vi "TimebaseSet.vi"(7 "参数查询(0)/设置(1)":bool, 8 "error in (no error)":errorcluster caption="错误输入（无错误）", 9 "设置参数":string, 10 "TIMEBASE命令子系统":string(combo), 11 "VISA资源名称":refnum<visa-resource-name>) -> (0 "error out":errorcluster caption="错误输出", 1 "查询返回字节数":u32, 2 "查询返回":string, 3 "VISA资源名称 2":refnum<visa-resource-name>)   [LabVIEW 2018]
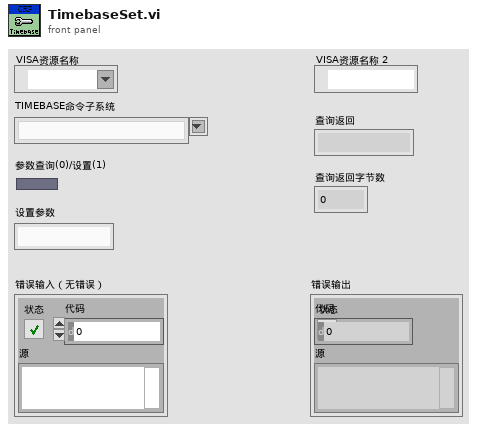
[diagram p1: front panel]
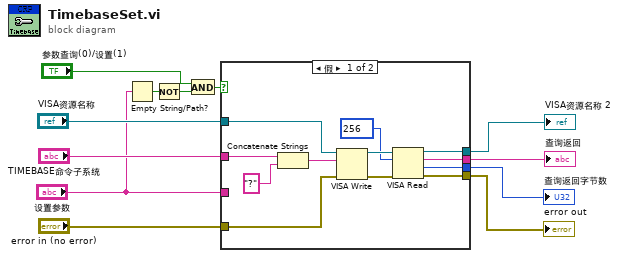
[diagram p0: block diagram]
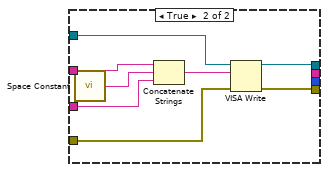
[diagram p2: hidden frame]
diagram:
  n1 = Empty String/Path?(string/path="设置参数") -> (empty?=w4:bool)
  n2 = Not(x=w4) -> (.not. x?=w1:bool)
  n3 = And(x="参数查询(0)/设置(1)", y=w1) -> (x .and. y?=w6:bool)
  n4 = case shown="假" w6 {
    tunnel: "设置参数" -> [_ w31]
    tunnel: "error in (no error)" -> [w14 w26]
    tunnel: [w20 w28] -> w11
    tunnel: [w19 _] -> w3
    tunnel: [w18 w29] -> w10
    tunnel: "TIMEBASE命令子系统" -> [w17 w30]
    tunnel: "VISA资源名称" -> [w15 w25]
    tunnel: [w13 _] -> w2
    frame False {
      n5 = Concatenate Strings(w17, "?") -> (w24:string)
      n6 = VISA Write(VISA resource name=w15, write buffer=w24, error in (no error)=w14) -> (VISA resource name out=w22:refnum<visa-resource-name>, error out=w23:errorcluster)  [unwired: 1 out]
      n7 = VISA Read(VISA resource name=w22, byte count=u32 256 ("字节总数"), error in (no error)=w23) -> (VISA resource name out=w18:refnum<visa-resource-name>, read buffer=w19:string, return count=w13:u32, error out=w20:errorcluster)
    }
    frame True {
      n8 = call <vilib>:"Space Constant.vi"() -> ("String"=w32:string)
      n9 = Concatenate Strings(w30, w32, w31) -> (w27:string)
      n10 = VISA Write(VISA resource name=w25, write buffer=w27, error in (no error)=w26) -> (VISA resource name out=w29:refnum<visa-resource-name>, error out=w28:errorcluster)  [unwired: 1 out]
    }
  }
  "error out" <- w11
  "VISA资源名称 2" <- w10
  "查询返回" <- w3
  "查询返回字节数" <- w2
